vi "Error Typedef.vi"() -> (0 "error in (no error)":errorcluster)   [LabVIEW 2017, in "WebServiceImporter.lvlib" / "Error Handling.lvlib"]
uses:
  <vilib>/Platform/WebService/Error Handling/Error Handling.lvlib
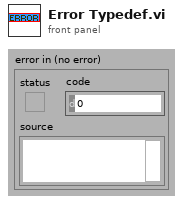
[diagram p1: front panel]
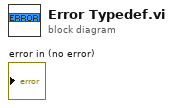
[diagram p0: block diagram]
diagram:
